vi "FunctionGen.vi"() -> ()   [LabVIEW 2019]
uses:
  4x7 segment controls/top-segment-f.ctl
  4x7 segment controls/left-segment-f.ctl
  4x7 segment controls/rigt-segment-f.ctl
  4x7 segment controls/mid-segment-f.ctl
  4x7 segment controls/bottom-segment-f.ctl
  4x7 segment controls/decimal-f.ctl
  4x7 segment controls/kHz-f.ctl
  4x7 segment controls/Hz-f.ctl
  type-f.ctl
  enum-f.ctl
  <vilib>/sound2/lvsound2.llb/Sound Output Task ID.ctl
  Globals/Global message.vi
  Globals/CH1.vi
  Globals/CH2.vi
  Globals/CH3.vi
  Globals/CH4.vi
  Globals/CH5.vi
  <vilib>/measure/NI_MABase.lvlib
  <vilib>/sound2/lvsound2.llb/Sampling Mode.ctl
  <vilib>/sound2/lvsound2.llb/Sound Data Format.ctl
  <vilib>/sound2/lvsound2.llb/Sound Output Write (DBL Single).vi
panel:
  in  "Output channel voltage":T1(ring)
  in  "Stop Button":bool
  in  "range":i32(knob) min=0 max=2 step=1 scale=0.0..2.0
  in  "fina":dbl(knob) caption="Фино" min=-0.5 max=0.5 step=0.01 scale=-0.5..0.5
  out "?":T10
  in  "pilest":bool
  in  "triagolen":bool
  in  "pravoagolen":bool
  in  "sinusoidalen":bool=TRUE
  in  "gruba":dbl(knob)=20.0 caption="Грубо" min=20.0 max=400.0 step=1.0 scale=20.0..400.0
  in  "amplituda":dbl(knob)=1.0 caption="Амплитуда" step=0.025 scale=0.0..10.0
  # "Тип на сигнал"
  # "Фреквенција"
  # "Опсег"
  # "4k"
  # "400"
  # "40k"
  # "ФУНКЦИСКИ ГЕНЕРАТОР"
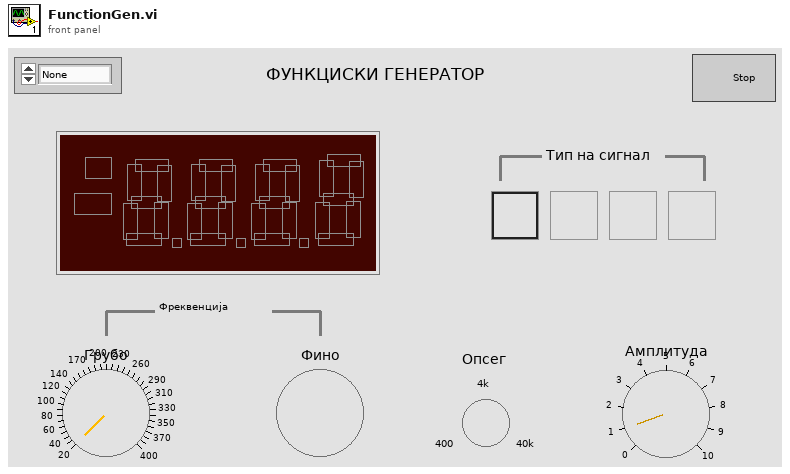
[diagram p1: front panel]
types:
  T1 = enum16{"None", "CH 1", "CH 2", "CH 3", "CH 4", "CH 5"}
  T2 = typedef "top-segment-f.ctl" = bool
  T3 = typedef "left-segment-f.ctl" = bool
  T4 = typedef "rigt-segment-f.ctl" = bool
  T5 = typedef "mid-segment-f.ctl" = bool
  T6 = typedef "bottom-segment-f.ctl" = bool
  T7 = typedef "decimal-f.ctl" = bool
  T8 = typedef "kHz-f.ctl" = bool
  T9 = typedef "Hz-f.ctl" = bool
  T10 = cluster{"1":cluster{"1":T2, "2":T3, "3":T4, "4":T5, "5":T3, "6":T4, "7":T6}, "2":cluster{"1":T2, "2":T3, "3":T4, "4":T5, "5":T3, "6":T4, "7":T6}, "3":cluster{"1":T2, "2":T3, "3":T4, "4":T5, "5":T3, "6":T4, "7":T6}, "4":cluster{"1":T2, "2":T3, "3":T4, "4":T5, "5":T3, "6":T4, "7":T6}, T7, T7, T7, T8, T9}
  T11 = typedef "enum-f.ctl" = enum16{"Inicijalizacija", "Generiranje"}
  T12 = typedef "type-f.ctl" = enum16{"Sinusoidalen", "Pravoagolen", "Triagolen", "Pilest"}
  T13 = typedef "Sound Data Format.ctl" = cluster{"sample rate (S/s)":dbl, "number of channels":i32, "bits per sample":i32}
  T14 = typedef "Sound Output Task ID.ctl" = u32
  T15 = typedef "Sampling Mode.ctl" = i32
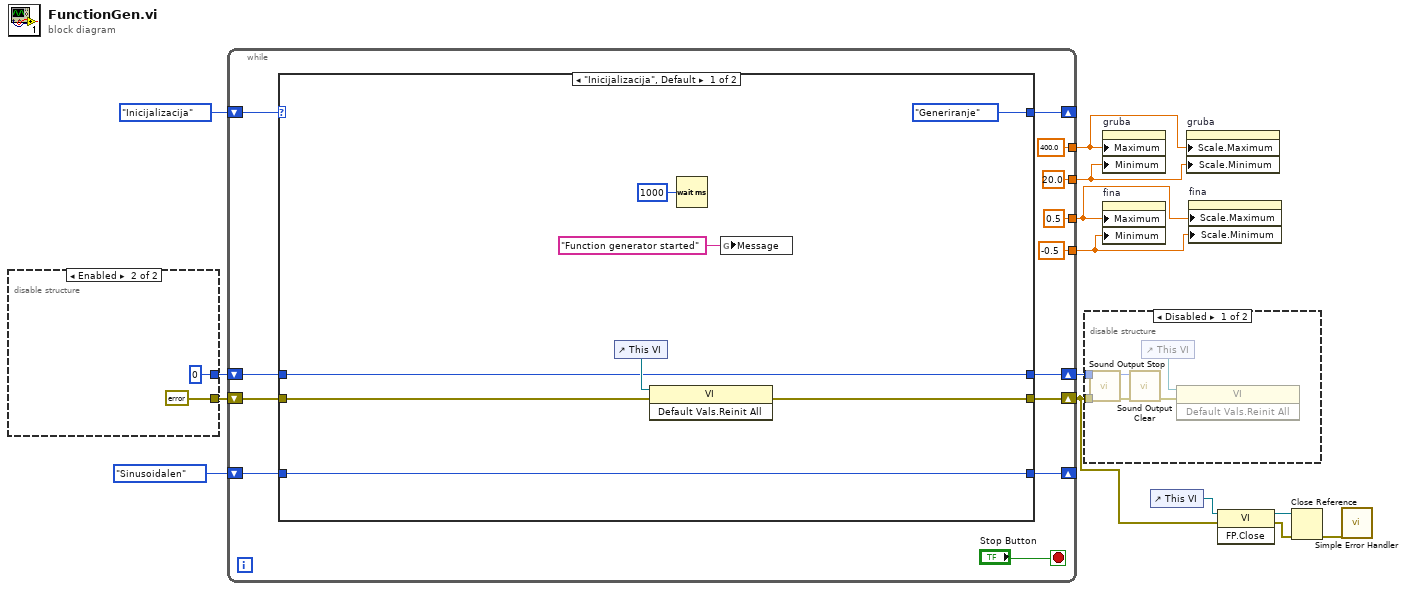
[diagram p0: block diagram]
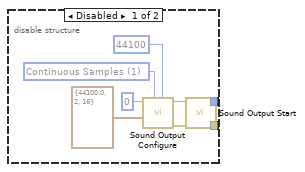
[diagram p2: hidden frame]
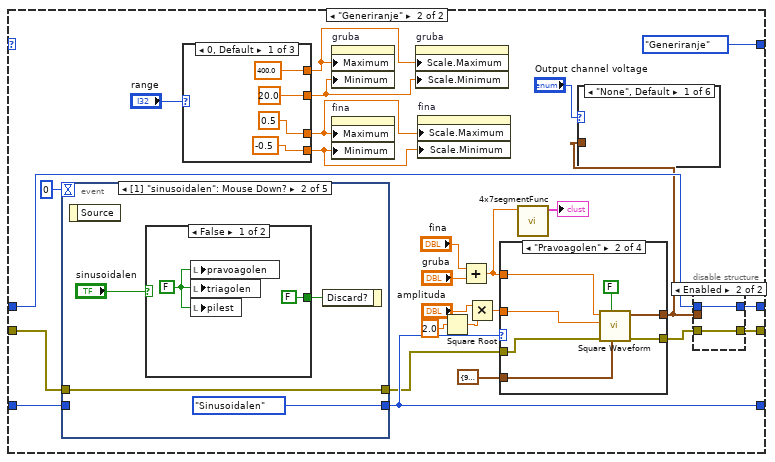
[diagram p4: hidden frame]
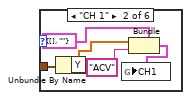
[diagram p5: hidden frame]
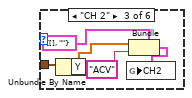
[diagram p6: hidden frame]
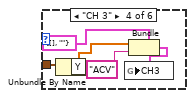
[diagram p7: hidden frame]
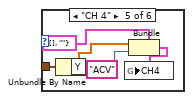
[diagram p8: hidden frame]
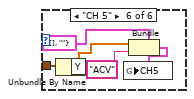
[diagram p9: hidden frame]
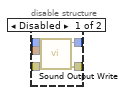
[diagram p10: hidden frame]
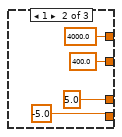
[diagram p11: hidden frame]
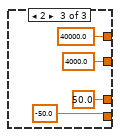
[diagram p12: hidden frame]
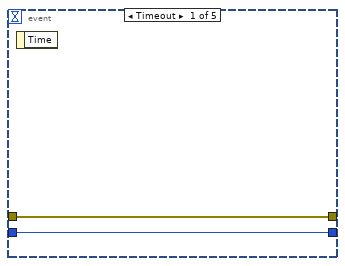
[diagram p13: hidden frame]
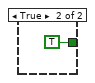
[diagram p14: hidden frame]
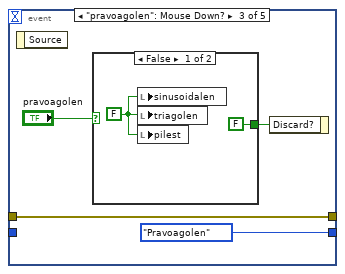
[diagram p15: hidden frame]
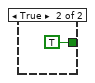
[diagram p16: hidden frame]
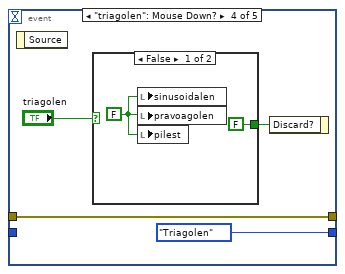
[diagram p17: hidden frame]
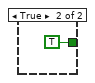
[diagram p18: hidden frame]
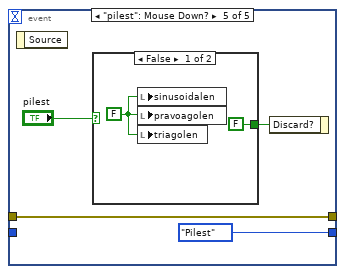
[diagram p19: hidden frame]
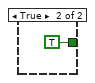
[diagram p20: hidden frame]
diagram:
  n1 = disable-structure shown="Enabled" {
    disable-tunnel: [w18 T14 0 ("task ID out")] -> w13
    disable-tunnel: [w17 errorcluster {"status"=FALSE, "code"=0, "source"=""} ("error out")] -> w12
    frame Disabled {
      w19 = T15 1 items=["Finite Samples", "Continuous Samples"] ("sample mode")
      n2 = call <vilib>:"Sound Output Configure.vi"("number of samples/ch"=44100, "sample mode"=w19, "sound format"=T13 {"sample rate (S/s)"=44100.0, "number of channels"=2, "bits per sample"=16}, "device ID"=u32 0) -> ("error out"=w16:errorcluster, "task ID"=w22:T14)  [unwired: 6 in]
      n3 = call <vilib>:"Sound Output Start.vi"("error in (no error)"=w16, "task ID"=w22) -> ("error out"=w17:errorcluster, "task ID out"=w18:T14)  [unwired: 8 in]
    }
    frame Enabled {
    }
  }
  n4 = while {
    shift-right: [w37] -> w14
    shift-left: w13 -> [w35]
    shift-right: [w36] -> w1
    shift-left: w12 -> [w34]
    shift-right: [w32] -> _
    shift-left: type-f."Sinusoidalen" ("Tip") -> [w33]
    shift-right: [w30] -> _
    shift-left: enum-f."Inicijalizacija" -> [w31]
    tunnel: [-0.5 ("Data Entry Limits:Maximum")] -> w9
    tunnel: [0.5 ("Data Entry Limits:Maximum")] -> w8
    tunnel: [20.0 ("Data Entry Limits:Maximum")] -> w7
    tunnel: [400.0 ("Data Entry Limits:Maximum")] -> w6
    stop <- "Stop Button" stop-if-true
    n5 = case shown="\"Inicijalizacija\", Default" w31 {
      tunnel: [w42 w71] -> w37
      tunnel: [w43 w70] -> w36
      tunnel: w35 -> [w42 w68]
      tunnel: w34 -> [w44 w67]
      tunnel: w33 -> [w41 w66]
      tunnel: [w41 w65] -> w32
      tunnel: [enum-f."Generiranje" enum-f."Generiranje"] -> w30
      frame "Inicijalizacija", Default {
        n6 = control-ref of="This VI"() -> (w45:refnum<vi>)
        n7 = invoke class="VI" method="Default Vals.Reinit All"(reference=w45, error in=w44) -> (error out=w43:errorcluster)  [unwired: 1 in, 2 out]
        n8 = Wait (ms)(milliseconds to wait=u32 1000) -> ()  [unwired: 1 out]
        n9 = global write "Global message.vi" "Message"("Function generator started") -> ()
      }
      frame "Generiranje" {
        n10 = event shown="[1] \"sinusoidalen\": Mouse Down?" {
          selector: _ -> [_ _ _ _ _]
          dyn-events: _ -> [_ _ _ _ _]
          timeout: 0 -> [_ _ _ _ _]
          tunnel: w67 -> [w117 w121 w128 w135 w142]
          tunnel: [w117 w121 w128 w135 w142] -> w54
          tunnel: w66 -> [w116 _ _ _ _]
          tunnel: [w116 type-f."Sinusoidalen" ("Tip") type-f."Pravoagolen" ("Tip") type-f."Triagolen" ("Tip") type-f."Pilest" ("Tip")] -> w65
          event Timeout {
            n11 = event-data() -> ()  [unwired: 1 in, 1 out]
          }
          event "sinusoidalen": Mouse Down? {
            n12 = event-data() -> ()  [unwired: 1 in, 1 out]
            n13 = case shown="False" "sinusoidalen" {
              tunnel: [FALSE TRUE] -> w119
              frame False {
                w123 = FALSE
                n14 = local write "pravoagolen"(w123) -> ()
                n15 = local write "triagolen"(w123) -> ()
                n16 = local write "pilest"(w123) -> ()
              }
              frame True {
              }
            }
            n17 = event-data("Discard?"=w119) -> ()  [unwired: 1 in, 1 out]
          }
          event "pravoagolen": Mouse Down? {
            n18 = event-data() -> ()  [unwired: 1 in, 1 out]
            n19 = case shown="False" "pravoagolen" {
              tunnel: [FALSE TRUE] -> w127
              frame False {
                w129 = FALSE
                n20 = local write "sinusoidalen"(w129) -> ()
                n21 = local write "triagolen"(w129) -> ()
                n22 = local write "pilest"(w129) -> ()
              }
              frame True {
              }
            }
            n23 = event-data("Discard?"=w127) -> ()  [unwired: 1 in, 1 out]
          }
          event "triagolen": Mouse Down? {
            n24 = event-data() -> ()  [unwired: 1 in, 1 out]
            n25 = case shown="False" "triagolen" {
              tunnel: [FALSE TRUE] -> w134
              frame False {
                w136 = FALSE
                n26 = local write "sinusoidalen"(w136) -> ()
                n27 = local write "pravoagolen"(w136) -> ()
                n28 = local write "pilest"(w136) -> ()
              }
              frame True {
              }
            }
            n29 = event-data("Discard?"=w134) -> ()  [unwired: 1 in, 1 out]
          }
          event "pilest": Mouse Down? {
            n30 = event-data() -> ()  [unwired: 1 in, 1 out]
            n31 = case shown="False" "pilest" {
              tunnel: [FALSE TRUE] -> w141
              frame False {
                w143 = FALSE
                n32 = local write "sinusoidalen"(w143) -> ()
                n33 = local write "pravoagolen"(w143) -> ()
                n34 = local write "triagolen"(w143) -> ()
              }
              frame True {
              }
            }
            n35 = event-data("Discard?"=w141) -> ()  [unwired: 1 in, 1 out]
          }
        }
        n36 = case shown="0, Default" "range" {
          tunnel: [400.0 ("Data Entry Limits:Maximum") 4000.0 ("Data Entry Limits:Maximum") 40000.0 ("Data Entry Limits:Maximum")] -> w56
          tunnel: [20.0 ("Data Entry Limits:Maximum") 400.0 ("Data Entry Limits:Maximum") 4000.0 ("Data Entry Limits:Maximum")] -> w55
          tunnel: [0.5 ("Data Entry Limits:Maximum") 5.0 ("Data Entry Limits:Maximum") 50.0 ("Data Entry Limits:Maximum")] -> w58
          tunnel: [-0.5 ("Data Entry Limits:Maximum") -5.0 ("Data Entry Limits:Maximum") -50.0 ("Data Entry Limits:Maximum")] -> w57
          frame 0, Default {
          }
          frame 1 {
          }
          frame 2 {
          }
        }
        n37 = property on="gruba" class="Knob (strict)"("Maximum"=w56, "Minimum"=w55) -> ()  [unwired: 2 in, 2 out]
        n38 = property on="fina" class="Knob (strict)"("Maximum"=w58, "Minimum"=w57) -> ()  [unwired: 2 in, 2 out]
        n39 = property on="gruba" class="Knob (strict)"("Scale.Maximum"=w56, "Scale.Minimum"=w55) -> ()  [unwired: 2 in, 2 out]
        n40 = property on="fina" class="Knob (strict)"("Scale.Maximum"=w58, "Scale.Minimum"=w57) -> ()  [unwired: 2 in, 2 out]
        n41 = Square Root(x=2.0) -> (sqrt(x)=w47:dbl)
        n42 = Add(x="fina", y="gruba") -> (x+y=w61:dbl)
        n43 = Multiply(x="amplituda", y=w47) -> (x*y=w49:dbl)
        n44 = case shown="\"Pravoagolen\"" w65 {
          tunnel: [w150 w157 w164 w171] -> w50
          tunnel: w61 -> [w151 w159 w166 w173]
          tunnel: w49 -> [w152 w158 w165 w172]
          tunnel: cluster{"Fs":dbl, "#s":dbl} {"Fs"=96000.0, "#s"=1000.0} ("sampling info") -> [w148 w156 w163 w169]
          tunnel: w54 -> [w147 w154 w161 w168]
          tunnel: [w146 w153 w160 w167] -> w53
          frame "Sinusoidalen", Default {
            n45 = call <vilib>:"Sine Waveform.vi"("sampling info"=w148, "reset signal"=FALSE, "error in (no error)"=w147, "amplitude"=w152, "frequency"=w151) -> ("error out"=w146:errorcluster, "signal out"=w150:waveform(dbl))  [unwired: 5 in]
          }
          frame "Pravoagolen" {
            n46 = call <vilib>:"Square Waveform.vi"("sampling info"=w156, "reset signal"=FALSE, "error in (no error)"=w154, "amplitude"=w158, "frequency"=w159) -> ("error out"=w153:errorcluster, "signal out"=w157:waveform(dbl))  [unwired: 5 in]
          }
          frame "Triagolen" {
            n47 = call <vilib>:"Triangle Waveform.vi"("sampling info"=w163, "reset signal"=FALSE, "error in (no error)"=w161, "amplitude"=w165, "frequency"=w166) -> ("error out"=w160:errorcluster, "signal out"=w164:waveform(dbl))  [unwired: 5 in]
          }
          frame "Pilest" {
            n48 = call <vilib>:"Sawtooth Waveform.vi"("sampling info"=w169, "reset signal"=FALSE, "error in (no error)"=w168, "amplitude"=w172, "frequency"=w173) -> ("error out"=w167:errorcluster, "signal out"=w171:waveform(dbl))  [unwired: 5 in]
          }
        }
        n49 = call "4x7segmentFunc.vi"("Numeric Control"=w61) -> (3:→"?":T10)  [unwired: 10 in]
        n50 = case shown="\"None\", Default" "Output channel voltage" {
          tunnel: w50 -> [_ w76 w78 w83 w88 w93]
          frame "None", Default {
          }
          frame "CH 1" {
            n51 = Unbundle By Name(w76) -> ("Y"=w74:dbl[])
            n52 = Bundle(cluster=cluster{"CH1 Array":dbl[], "CH1 Message":string} {"CH1 Array"=[], "CH1 Message"=""} ("CH1"), "CH1 Array"=w74, "CH1 Message"="ACV") -> (w73:cluster{"CH1 Array":dbl[], "CH1 Message":string})
            n53 = global write "CH1.vi" "CH1"(w73) -> ()
          }
          frame "CH 2" {
            n54 = Unbundle By Name(w78) -> ("Y"=w80:dbl[])
            n55 = Bundle(cluster=cluster{"CH1 Array":dbl[], "CH1 Message":string} {"CH1 Array"=[], "CH1 Message"=""} ("CH1"), "CH1 Array"=w80, "CH1 Message"="ACV") -> (w77:cluster{"CH1 Array":dbl[], "CH1 Message":string})
            n56 = global write "CH2.vi" "CH2"(w77) -> ()
          }
          frame "CH 3" {
            n57 = Unbundle By Name(w83) -> ("Y"=w85:dbl[])
            n58 = Bundle(cluster=cluster{"CH1 Array":dbl[], "CH1 Message":string} {"CH1 Array"=[], "CH1 Message"=""} ("CH1"), "CH1 Array"=w85, "CH1 Message"="ACV") -> (w82:cluster{"CH1 Array":dbl[], "CH1 Message":string})
            n59 = global write "CH3.vi" "CH3"(w82) -> ()
          }
          frame "CH 4" {
            n60 = Unbundle By Name(w88) -> ("Y"=w90:dbl[])
            n61 = Bundle(cluster=cluster{"CH1 Array":dbl[], "CH1 Message":string} {"CH1 Array"=[], "CH1 Message"=""} ("CH1"), "CH1 Array"=w90, "CH1 Message"="ACV") -> (w87:cluster{"CH1 Array":dbl[], "CH1 Message":string})
            n62 = global write "CH4.vi" "CH4"(w87) -> ()
          }
          frame "CH 5" {
            n63 = Unbundle By Name(w93) -> ("Y"=w95:dbl[])
            n64 = Bundle(cluster=cluster{"CH1 Array":dbl[], "CH1 Message":string} {"CH1 Array"=[], "CH1 Message"=""} ("CH1"), "CH1 Array"=w95, "CH1 Message"="ACV") -> (w92:cluster{"CH1 Array":dbl[], "CH1 Message":string})
            n65 = global write "CH5.vi" "CH5"(w92) -> ()
          }
        }
        n66 = disable-structure shown="Enabled" {
          disable-tunnel: w50 -> [w101 _]
          disable-tunnel: [w100 w102] -> w71
          disable-tunnel: [w99 w103] -> w70
          disable-tunnel: w68 -> [w98 w102]
          disable-tunnel: w53 -> [w97 w103]
          frame Disabled {
            n67 = call-poly <vilib>:"Sound Output Write.vi"("error in (no error)"=w97, "data"=w101, "task ID"=w98) -> ("error out"=w99:errorcluster, "task ID out"=w100:T14)  [unwired: 7 in]
          }
          frame Enabled {
          }
        }
      }
    }
  }
  n68 = disable-structure shown="Disabled" {
    disable-tunnel: w14 -> [w177 _]
    disable-tunnel: w1 -> [w176 _]
    frame Disabled {
      n69 = call <vilib>:"Sound Output Stop.vi"("error in (no error)"=w176, "task ID"=w177) -> ("error out"=w178:errorcluster, "task ID out"=w179:T14)  [unwired: 8 in]
      n70 = call <vilib>:"Sound Output Clear.vi"("error in (no error)"=w178, "task ID"=w179) -> ("error out"=w174:errorcluster)  [unwired: 9 in]
      n71 = control-ref of="This VI"() -> (w175:refnum<vi>)
      n72 = invoke class="VI" method="Default Vals.Reinit All"(reference=w175, error in=w174) -> ()  [unwired: 1 in, 3 out]
    }
    frame Enabled {
    }
  }
  n73 = property on="gruba" class="Knob (strict)"("Maximum"=w6, "Minimum"=w7) -> ()  [unwired: 2 in, 2 out]
  n74 = property on="fina" class="Knob (strict)"("Maximum"=w8, "Minimum"=w9) -> ()  [unwired: 2 in, 2 out]
  n75 = control-ref of="This VI"() -> (w4:refnum<vi>)
  n76 = property on="gruba" class="Knob (strict)"("Scale.Maximum"=w6, "Scale.Minimum"=w7) -> ()  [unwired: 2 in, 2 out]
  n77 = property on="fina" class="Knob (strict)"("Scale.Maximum"=w8, "Scale.Minimum"=w9) -> ()  [unwired: 2 in, 2 out]
  n78 = invoke class="VI" method="FP.Close"(reference=w4, error in=w1) -> (reference out=w2:refnum<vi>, error out=w3:errorcluster)  [unwired: 1 in, 1 out]
  n79 = Close Reference(reference=w2, error in (no error)=w3) -> (error out=w5:errorcluster)
  n80 = call <vilib>:"Simple Error Handler.vi"("error in (no error)"=w5) -> ()  [unwired: 4 in, 5 out]
